vi "getSerializedData.vi"(0 "reference":refnum<class "CallNode.lvclass">, 5 "error in (no error)":errorcluster) -> (14 "reference out":refnum<class "CallNode.lvclass">, 15 "parent":refnum<class "AbstractNode.lvclass">, 16 "children":refnum<class "AbstractNode.lvclass">[](array[class]), 17 "xmlOut":string, 19 "error out":errorcluster)   [LabVIEW 2016, in "CallNode.lvclass"]
uses:
  <resource>/Framework/Providers/Open_GDS/UML/CallNode_class/CallNode.lvclass
  C:/Program Files (x86)/National Instruments/LabVIEW 2016/resource/Framework/Providers/Open_GDS/UML/RectangularNode_class/RectangularNode.lvclass
  C:/Program Files (x86)/National Instruments/LabVIEW 2016/resource/Framework/Providers/Open_GDS/UML/AbstractNode_class/AbstractNode.lvclass
  <resource>/Framework/Providers/Open_GDS/UML/AbstractNode_class/AbstractNode.lvclass
  <resource>/Framework/Providers/Open_GDS/UML/General/Rectangle/Rectangle Rectangle2D.ctl
  <resource>/Framework/Providers/Open_GDS/UML/RectangularNode_class/RectangularNode.lvclass
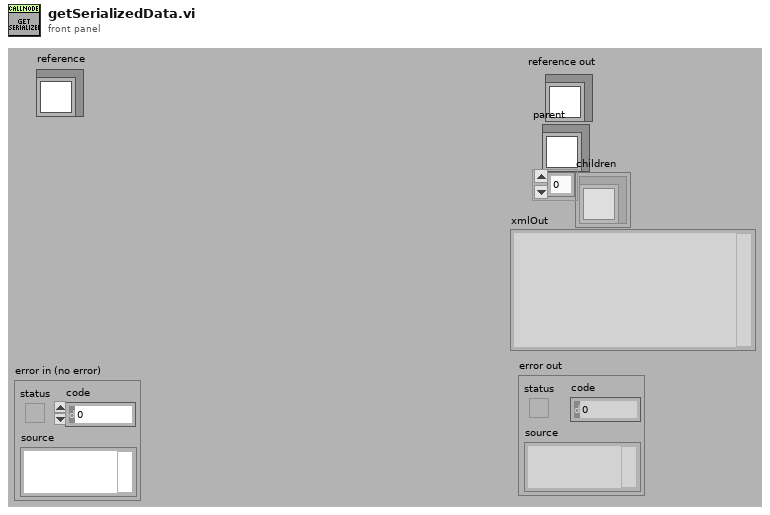
[diagram p1: front panel]
types:
  T1 = typedef "Rectangle Rectangle2D.ctl" = cluster{"x":dbl, "y":dbl, "width":dbl, "height":dbl}
  T2 = cluster{"Base class":cluster{"Base class":cluster{"parent":refnum<k1>, "children":refnum<k1>[]}, "bounds":T1}, "objectCallNodeRef":refnum<k1>, "signaled":bool, "openBottom":bool, "DEFAULT_WIDTH":i32, "DEFAULT_HEIGHT":i32, "CALL_YGAP":i32}
  T3 = typedef "CallNode.lvclass/ObjectAttributes.ctl" = cluster{"objectCallNodeRef":refnum<class "AbstractNode.lvclass">, "signaled":bool, "openBottom":bool, "DEFAULT_WIDTH":i32, "DEFAULT_HEIGHT":i32, "CALL_YGAP":i32}
  T4 = typedef "RectangularNode.lvclass/ObjectAttributes.ctl" = cluster{"bounds":T1}
  T5 = typedef "AbstractNode.lvclass/ObjectAttributes.ctl" = cluster{"parent":refnum<class "AbstractNode.lvclass">, "children":refnum<class "AbstractNode.lvclass">[], "Hidden":bool}
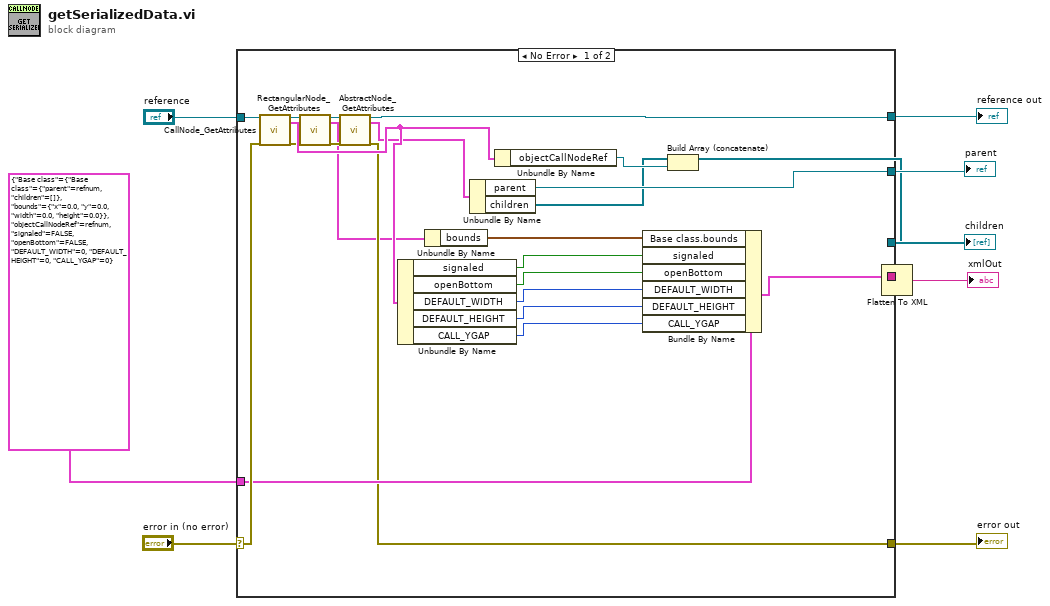
[diagram p0: block diagram]
diagram:
  n1 = case shown="No Error" "error in (no error)" {
    selector: "error in (no error)" -> [w32 w33]
    tunnel: "reference" -> [w31 w34]
    tunnel: [w12 w33] -> w6
    tunnel: [w11 w34] -> w5
    tunnel: [w30 _] -> w4
    tunnel: [w27 _] -> w3
    tunnel: [w29 _] -> w2
    tunnel: T2 {"Base class"={"Base class"={"parent"=refnum, "children"=[]}, "bounds"={"x"=0.0, "y"=0.0, "width"=0.0, "height"=0.0}}, "objectCallNodeRef"=refnum, "signaled"=FALSE, "openBottom"=FALSE, "DEFAULT_WIDTH"=0, "DEFAULT_HEIGHT"=0, "CALL_YGAP"=0} ("Attributes") -> [w25 _]
    frame No Error {
      n2 = call <resource>:"CallNode_GetAttributes.vi"("reference in"=w31, "error in (no error)"=w32) -> ("reference out"=w16:refnum<class "CallNode.lvclass">, "Data"=w17:T3, "error out"=w15:errorcluster)  [unwired: 1 in, 14 out]
      n3 = call <resource>:"RectangularNode_GetAttributes.vi"("reference in"=w16, "error in (no error)"=w15) -> ("reference out"=w14:refnum<class "CallNode.lvclass">, "Data"=w9:T4, "error out"=w13:errorcluster)  [unwired: 14 in, 1 out]
      n4 = call <resource>:"AbstractNode_GetAttributes.vi"("reference in"=w14, "error in (no error)"=w13) -> ("reference out"=w11:refnum<class "CallNode.lvclass">, "Data"=w10:T5, "error out"=w12:errorcluster)  [unwired: 14 in, 1 out]
      n5 = Unbundle By Name(w17) -> ("signaled"=w23:bool, "openBottom"=w22:bool, "DEFAULT_WIDTH"=w21:i32, "DEFAULT_HEIGHT"=w20:i32, "CALL_YGAP"=w19:i32)
      n6 = Unbundle By Name(w9) -> ("bounds"=w24:T1)
      n7 = Unbundle By Name(w10) -> ("parent"=w30:refnum<class "AbstractNode.lvclass">, "children"=w26:refnum<class "AbstractNode.lvclass">[])
      n8 = Unbundle By Name(w17) -> ("objectCallNodeRef"=w28:refnum<class "AbstractNode.lvclass">)
      n9 = Bundle By Name(cluster=w25, "Base class.bounds"=w24, "signaled"=w23, "openBottom"=w22, "DEFAULT_WIDTH"=w21, "DEFAULT_HEIGHT"=w20, "CALL_YGAP"=w19) -> (w18:T2)
      n10 = Build Array (concatenate)(w26, w28) -> (w27:refnum<class "AbstractNode.lvclass">[])
      n11 = Flatten To XML(anything=w18) -> (xml string=w29:string)
    }
    frame Error {
    }
  }
  "reference out" <- w5
  "error out" <- w6
  "children" <- w3
  "parent" <- w4
  "xmlOut" <- w2
